vi "read 8b u64 number.vi"(8 "error in (no error)":errorcluster, 11 "TCP Network Connection in":refnum<k5>) -> (0 "error out":errorcluster, 2 "number":u64, 3 "TCP Network Connection out":refnum<k5>)   [LabVIEW 2020]
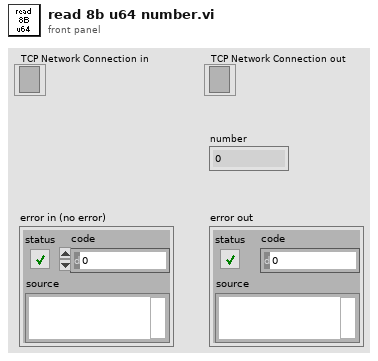
[diagram p1: front panel]
types:
  T1 = enum16{"big-endian, network order", "native, host order", "little-endian"}
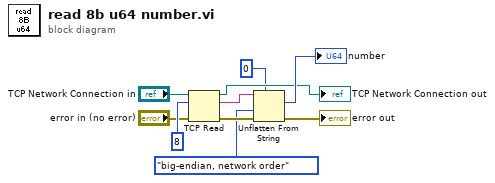
[diagram p0: block diagram]
diagram:
  n1 = TCP Read(connection ID="TCP Network Connection in", bytes to read=8, error in (no error)="error in (no error)") -> (connection ID out=→"TCP Network Connection out":refnum<k5>, data out=w7:string, error out=w6:errorcluster)  [unwired: 2 in]
  n2 = Unflatten From String(type=u64 0 ("bytes to read"), binary string=w7, byte order (0:big-endian, network order)=T1."big-endian, network order", error in (no error)=w6) -> (value=→"number":u64, error out=→"error out":errorcluster)  [unwired: 1 in, 1 out]
